vi "Get HTTP Port.vi"(8 "error in (no error)":errorcluster, 11 "Node in":refnum<class "Node Config.lvclass">) -> (0 "error out":errorcluster, 2 "HTTP Port":u16, 3 "Node out":refnum<class "Node Config.lvclass">)   [LabVIEW 2020, in "Vecto.lvlib" / "Node Config.lvclass"]
uses:
  Node Config.lvclass
  Node Config.lvclass/Node Config.ctl
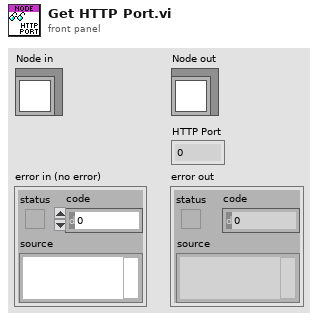
[diagram p1: front panel]
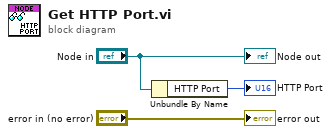
[diagram p0: block diagram]
diagram:
  n1 = Unbundle By Name("Node in") -> ("HTTP Port"=→"HTTP Port":u16)
  "error out" <- "error in (no error)"
  "Node out" <- "Node in"
